vi "PlotMultipleXYCurves.vi"() -> ()   [LabVIEW 2015]
panel:
  out "XY图":cluster{"X":dbl[], "Y":dbl[]}[](graph)
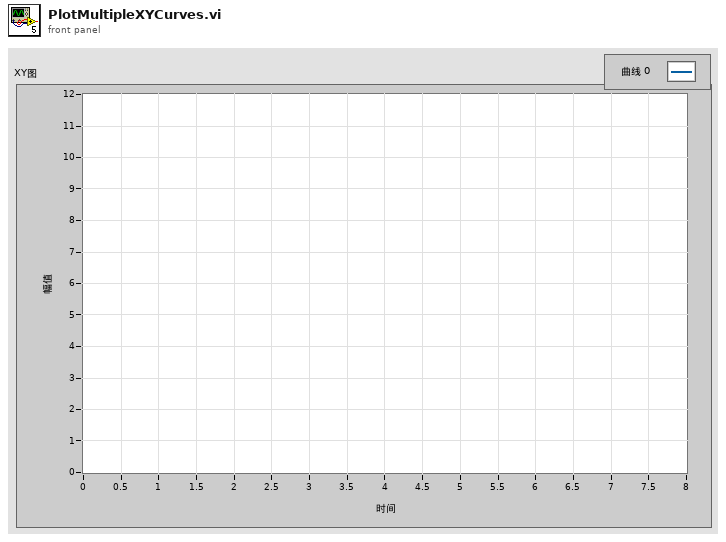
[diagram p1: front panel]
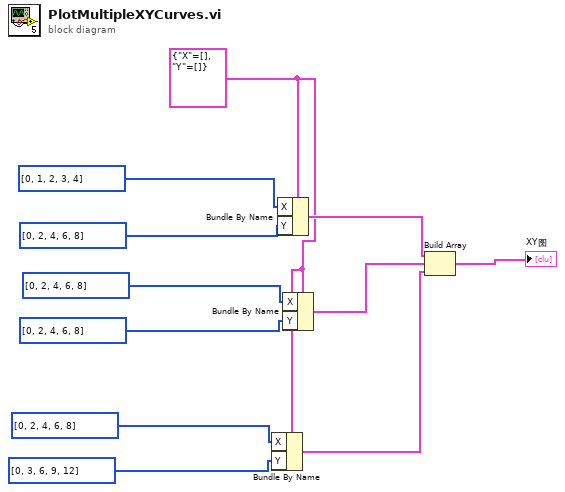
[diagram p0: block diagram]
diagram:
  w3 = cluster{"X":dbl[], "Y":dbl[]} {"X"=[], "Y"=[]} ("输入簇")
  n1 = Bundle By Name(cluster=w3, "X"=i32[] [0, 2, 4, 6, 8], "Y"=i32[] [0, 3, 6, 9, 12]) -> (w1:cluster{"X":dbl[], "Y":dbl[]})
  n2 = Bundle By Name(cluster=w3, "X"=i32[] [0, 1, 2, 3, 4], "Y"=i32[] [0, 2, 4, 6, 8]) -> (w7:cluster{"X":dbl[], "Y":dbl[]})
  n3 = Bundle By Name(cluster=w3, "X"=i32[] [0, 2, 4, 6, 8], "Y"=i32[] [0, 2, 4, 6, 8]) -> (w2:cluster{"X":dbl[], "Y":dbl[]})
  n4 = Build Array(w7, w2, w1) -> (→"XY图":cluster{"X":dbl[], "Y":dbl[]}[])
